vi "Created.vi"(6 "Created Alias":string, 7 "jettl in":refnum<class "jettl.lvclass">, 8 "Priority?":bool, 9 "Msg Strategy":refnum<class "Msg Strategy.lvclass">, 10 "Addresses DVR":refnum<data-value>) -> (5 "jettl out":refnum<class "jettl.lvclass">)   [LabVIEW 2021, in "jettl.lvlib" / "Addresses.lvlib"]
uses:
  Addresses.lvlib
  Error/Error.lvlib
  jettl/jettl.lvclass
  Msg Type Strategy/Msg Type Strategy/Msg Type Strategy.lvclass
  Msg Strategy/Msg Strategy.lvclass
  Addresses/Addresses.lvclass
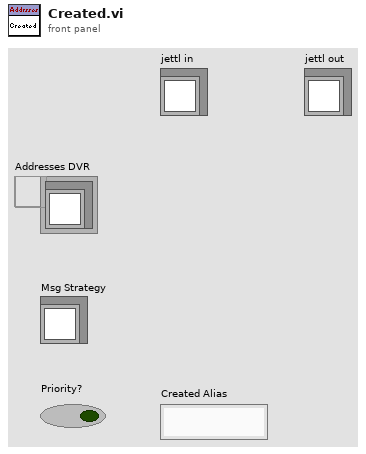
[diagram p1: front panel]
types:
  T1 = typedef "jettl.lvlib/Addresses.lvlib/Created.ctl" = map{string, refnum<class "Msg Type Strategy.lvclass">}
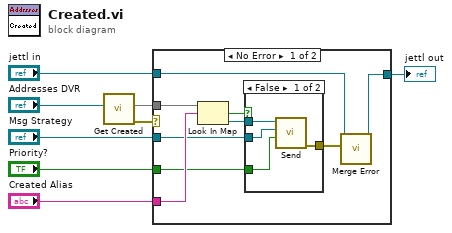
[diagram p0: block diagram]
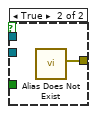
[diagram p2: hidden frame]
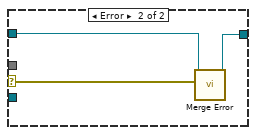
[diagram p3: hidden frame]
diagram:
  n1 = call "Get Created.vi"("Addresses DVR"="Addresses DVR") -> ("error out"=w1:errorcluster, "Created"=w3:T1)  [unwired: 9 in]
  n2 = case shown="No Error" w1 {
    selector: w1 -> [_ w23]
    tunnel: "Created Alias" -> [w14 _]
    tunnel: "Priority?" -> [w13 _]
    tunnel: "Msg Strategy" -> [w12 _]
    tunnel: [w11 w24] -> w5
    tunnel: "jettl in" -> [w10 w25]
    tunnel: w3 -> [w9 _]
    frame No Error {
      n3 = Look In Map(map=w9, key=w14) -> (key not found?=w16:bool, value=w17:refnum<class "Msg Type Strategy.lvclass">)  [unwired: 1 in]
      n4 = case shown="False" w16 {
        tunnel: [w21 w22] -> w15
        tunnel: w13 -> [w18 _]
        tunnel: w12 -> [w19 _]
        tunnel: w17 -> [w20 _]
        frame False {
          n5 = call-dynamic "Send.vi"("Priority?"=w18, "Msg Strategy"=w19, "Msg Type Strategy in"=w20) -> ("error out"=w21:errorcluster)  [unwired: 8 in]
        }
        frame True {
          n6 = call "Alias Does Not Exist.vi"() -> ("Error"=w22:errorcluster)  [unwired: 11 in]
        }
      }
      n7 = call-dynamic "Merge Error.vi"("Error"=w15, "Merge Error in"=w10) -> ("Merge Error out"=w11:refnum<class "jettl.lvclass">)  [unwired: 9 in]
    }
    frame Error {
      n8 = call-dynamic "Merge Error.vi"("Error"=w23, "Merge Error in"=w25) -> ("Merge Error out"=w24:refnum<class "jettl.lvclass">)  [unwired: 9 in]
    }
  }
  "jettl out" <- w5
